vi "PID Integrate Vector.vi"(6 "dt":dbl, 9 "Array length":i32, 10 "Index array":i32[](array[numeric]), 11 "Integrate array":dbl[](array[numeric])) -> (2 "Timed integration":dbl[](array[numeric]), 3 "Time point results":dbl[](array[numeric]))   [LabVIEW 2020, in "NI_PID_autopid.lvlib"]
uses:
  <vilib>/addons/control/pid/NI_PID_autopid.lvlib
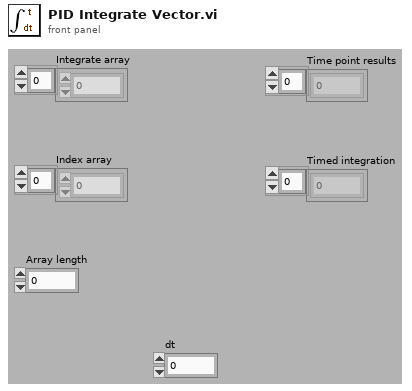
[diagram p1: front panel]
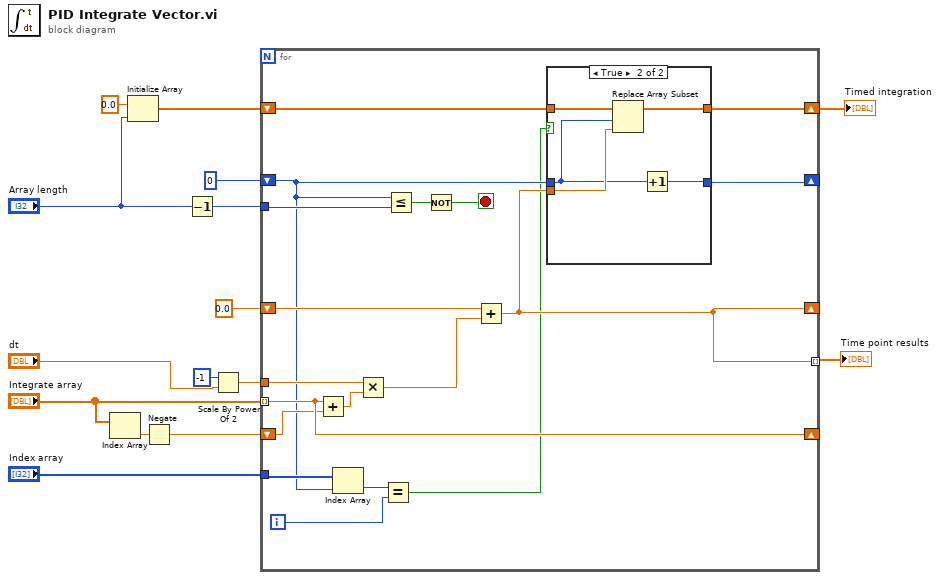
[diagram p0: block diagram]
diagram:
  n1 = Index Array(array="Integrate array") -> (element=w11:dbl)  [unwired: 1 in]
  n2 = Initialize Array(0.0 ("element"), "Array length") -> (w1:dbl[])
  n3 = Negate(x=w11) -> (-x=w9:dbl)
  n4 = Decrement(x="Array length") -> (x-1=w10:i32)
  n5 = Scale By Power Of 2(n=-1, x="dt") -> (x*2^n=w5:dbl)
  n6 = for {
    tunnel: "Integrate array" -> [w30] mode=indexing
    shift-right: [w26] -> _
    shift-left: 0.0 -> [w33]
    tunnel: [w26] -> w15 mode=indexing
    shift-right: [w23] -> _
    shift-left: 0 ("index") -> [w19]
    tunnel: w10 -> [w31]
    shift-right: [w30] -> _
    shift-left: w9 -> [w29]
    shift-right: [w24] -> w8
    shift-left: w1 -> [w25]
    tunnel: w5 -> [w22]
    tunnel: "Index array" -> [w20]
    i -> [w17]
    stop <- w32 stop-if-true
    n7 = Add(x=w30, y=w29) -> (x+y=w28:dbl)
    n8 = Index Array(array=w20, index=w19) -> (element=w18:i32)
    n9 = Multiply(x=w22, y=w28) -> (x*y=w21:dbl)
    n10 = Equal?(x=w18, y=w17) -> (x = y?=w16:bool)
    n11 = Less Or Equal?(x=w19, y=w31) -> (x <= y?=w27:bool)
    n12 = Not(x=w27) -> (.not. x?=w32:bool)
    n13 = Add(x=w33, y=w21) -> (x+y=w26:dbl)
    n14 = case shown="True" w16 {
      tunnel: w26 -> [_ w39]
      tunnel: w25 -> [w35 w40]
      tunnel: w19 -> [w34 w37]
      tunnel: [w35 w38] -> w24
      tunnel: [w34 w36] -> w23
      frame False {
      }
      frame True {
        n15 = Replace Array Subset(array=w40, new element=w39, index=w37) -> (w38:dbl[])
        n16 = Increment(x=w37) -> (x+1=w36:i32)
      }
    }
  }
  "Time point results" <- w15
  "Timed integration" <- w8
